vi "KeDSO Initialize Virtual Channels.vi"(8 "error in":errorcluster, 10 "Reset (True)":bool=TRUE, 11 "keysight dso":T1={"VISA"="", "channels"=[], "bw limit [Hz]"=0.0, "resolution"=enum."Basic", "trig noise reject"=enum."Normal", "N"=0, "trigger config"={"trigger source"=enum."Immediate", "trigger slope"=enum."Negative", "level [V]"=0.0, "hysteresis [V]"=0.001, "pre-trig [%]"=50}, "fs [Hz]"=0.0, "timeout stop"=timestamp(0 s since 1904-01-01), "waiting for opc"=FALSE, "fetch offset [smpl]"=0, "abs timestamp"=timestamp(0 s since 1904-01-01), "ranges [V]"=[], "decimation"=0.0, "ext ref"=FALSE, "emulate aperture"=FALSE, "model"=enum."DSO91304"} {"bw limit [Hz]" format="%#_6p"; "channels"."Offset [V]" format="%#_6p"; "channels"."Range [Vpk]" min=0.0 format="%#_6p"; "channels"."Channel" min=1}) -> (0 "error out":errorcluster, 2 "channel ids":string[](array[string]), 3 "keysight dso out":T1={"VISA"="", "channels"=[], "bw limit [Hz]"=0.0, "resolution"=enum."Basic", "trig noise reject"=enum."Normal", "N"=0, "trigger config"={"trigger source"=enum."Immediate", "trigger slope"=enum."Negative", "level [V]"=0.0, "hysteresis [V]"=0.001, "pre-trig [%]"=50}, "fs [Hz]"=0.0, "timeout stop"=timestamp(0 s since 1904-01-01), "waiting for opc"=FALSE, "fetch offset [smpl]"=0, "abs timestamp"=timestamp(0 s since 1904-01-01), "ranges [V]"=[], "decimation"=0.0, "ext ref"=FALSE, "emulate aperture"=FALSE, "model"=enum."DSO91304"} {"bw limit [Hz]" format="%#_6p"; "channels"."Offset [V]" format="%#_6p"; "channels"."Range [Vpk]" min=0.0 format="%#_6p"; "channels"."Channel" min=1})   [LabVIEW 2020]
doc: "Initializes virtual channels of Keysight DSOs according to keysight session data."
uses:
  KeDSO session.ctl
  KeDSO Virtual Channel.ctl
  KeDSO High Resolution Mode.ctl
  KeDSO Trigger Setup.ctl
  KeDSO Trigger Source.ctl
  Agilent 90000 Series.lvlib
  Public/Utility/DSO type.ctl
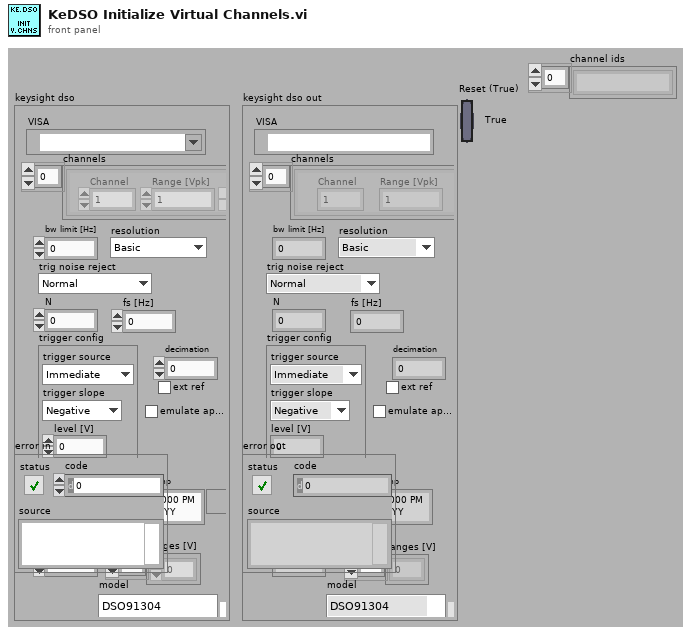
[diagram p1: front panel]
types:
  T1 = typedef "KeDSO session.ctl" = cluster{"VISA":refnum<visa-resource-name>, "channels":T2[], "bw limit [Hz]":dbl, "resolution":T3, "trig noise reject":enum16{"Normal", "High Sensitivity"}, "N":i64, "trigger config":T4, "fs [Hz]":dbl, "timeout stop":timestamp, "waiting for opc":bool, "fetch offset [smpl]":i64, "abs timestamp":timestamp, "ranges [V]":dbl[], "decimation":dbl, "ext ref":bool, "emulate aperture":bool, "model":T6}
  T2 = typedef "KeDSO Virtual Channel.ctl" = cluster{"Channel":i32, "Range [Vpk]":dbl, "btn clr":bool, "btn up":bool, "btn down":bool, "Offset [V]":dbl, "Coupling":enum16{"DC", "DC50", "AC", "LFR1"}, "bw limit enab":bool}
  T3 = typedef "KeDSO High Resolution Mode.ctl" = enum16{"Basic", "High-res AUTO", "Min. 9-bits", "Min. 10-bits", "Min. 11-bits", "Min. 12-bits", "Fixed 11-bits", "Fixed 12-bits", "Fixed 13-bits", "Fixed 14-bits", "Fixed 15-bits", "Fixed 16-bits"}
  T4 = typedef "KeDSO Trigger Setup.ctl" = cluster{"trigger source":T5, "trigger slope":enum16{"Negative", "Positive", "Either"}, "level [V]":dbl, "hysteresis [V]":dbl, "pre-trig [%]":i32}
  T5 = typedef "KeDSO Trigger Source.ctl" = enum16{"Immediate", "Level", "AUX"}
  T6 = typedef "Agilent 90000 Series.lvlib/DSO type.ctl" = enum16{"DSO91304", "DSO91204", "DSO90804", "DSO90604", "DSO90404", "DSO90254", "DSA91304", "DSA91204", "DSA90804", "DSA90604", "DSA90404", "DSA90254", "DSO9104", "DSO9254", "DSO9404", "MSO9104", "MSO9254", "MSO9404", "MSO9064", "DSO9064", "DSOX91604", "DSOX92004", "DSOX92504", "DSOX92804", "DSOX93204", "DSO93004", "DSO9024H", "DSO9054H", "DSO9104H", "DSO9204H", "DSOS054A", "DSOS104A", "DSOS204A", "DSOS254A", "DSOS404A", "DSOS604A", "DSOS804A", "MSOS054A", "MSOS104A", "MSOS204A", "MSOS254A", "MSOS404A", "MSOS604A", "MSOS804A", "DSAX96204Q", "DSOX96204Q", "DSAX95004Q", "DSOX95004Q", "DSAX93304Q", "DSOX93304Q", "DSAX92504Q", "DSOX92504Q", "DSAX92004Q", "DSOX92004Q"}
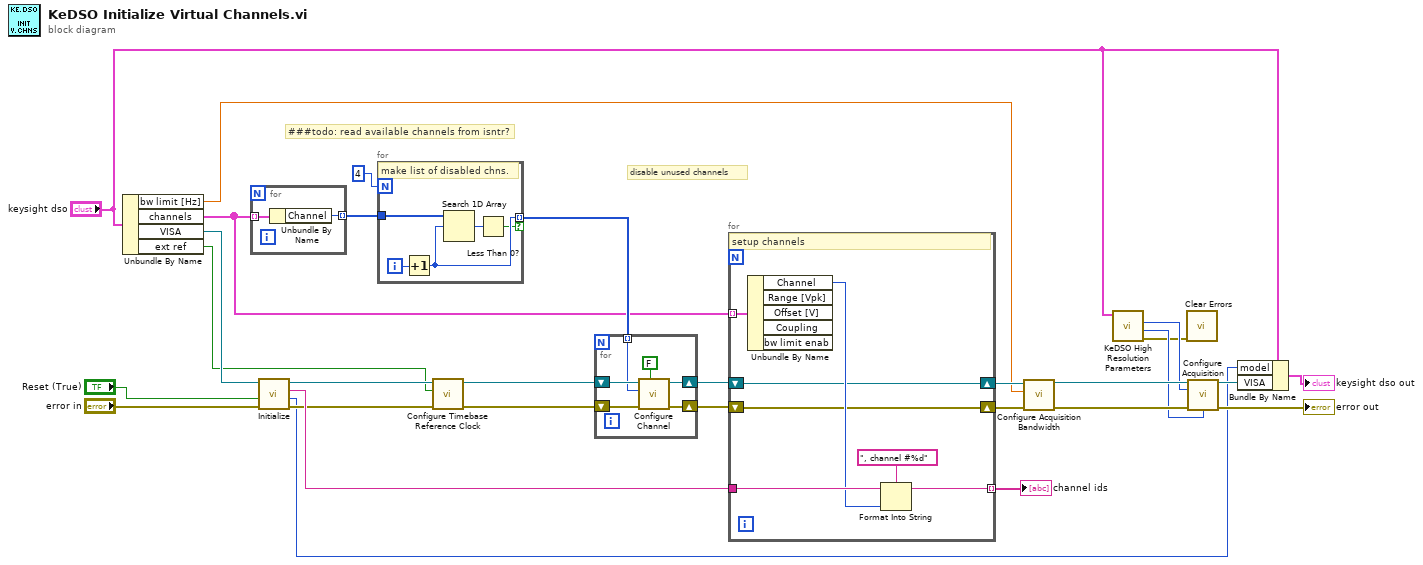
[diagram p0: block diagram]
diagram:
  # "disable unused channels"
  # "###todo: read available channels from isntr?"
  n1 = Unbundle By Name("keysight dso") -> ("bw limit [Hz]"=w18:dbl, "channels"=w21:T2[], "VISA"=w28:refnum<visa-resource-name>, "ext ref"=w2:bool)
  n2 = for {
    tunnel: w21 -> [w31] mode=indexing
    tunnel: [w30] -> w25 mode=indexing
    n3 = Unbundle By Name(w31) -> ("Channel"=w30:i32)
  }
  n4 = call "Initialize.vi"("error in (no error)"="error in", "Reset (True)"="Reset (True)", "VISA resource name"=w28) -> ("error out"=w6:errorcluster, "model"=w1:T6, "idn string"=w16:string, "VISA resource name out"=w5:refnum<visa-resource-name>)  [unwired: 5 in]
  n5 = for {
    N: 4 -> [_]
    tunnel: w25 -> [w36]
    tunnel: [w34] -> w24 mode=indexing if=w32
    i -> [w35]
    # "make list of disabled chns."
    n6 = Increment(x=w35) -> (x+1=w34:i32)
    n7 = Search 1D Array(1D array=w36, element=w34) -> (index of element=w33:i32)  [unwired: 1 in]
    n8 = Less Than 0?(x=w33) -> (x < 0?=w32:bool)
  }
  n9 = call "Configure Timebase Reference Clock.vi"("error in (no error)"=w6, "use ext ref (F: local)"=w2, "VISA resource name"=w5) -> ("error out"=w4:errorcluster, "VISA resource name out"=w3:refnum<visa-resource-name>)  [unwired: 7 in]
  n10 = for {
    shift-right: [w37] -> w22
    shift-left: w3 -> [w41]
    shift-right: [w38] -> w23
    shift-left: w4 -> [w42]
    tunnel: w24 -> [w39] mode=indexing
    n11 = call "Configure Channel.vi"("Enable Channel (T: Enable)"=FALSE, "error in (no error)"=w42, "Channel (1: Channel 1)"=w39, "VISA resource name"=w41) -> ("error out"=w38:errorcluster, "VISA resource name out"=w37:refnum<visa-resource-name>)  [unwired: 6 in]
  }
  n12 = for {
    shift-right: [w44] -> w19
    shift-left: w22 -> [w44]
    shift-right: [w43] -> w20
    shift-left: w23 -> [w43]
    tunnel: w21 -> [w49] mode=indexing
    tunnel: w16 -> [w48]
    tunnel: [w45] -> w15 mode=indexing
    # "setup channels"
    n13 = Unbundle By Name(w49) -> ("Channel"=w46:i32)  [unwired: 4 out]
    n14 = Format Into String(format string=", channel #%d", initial string=w48, w46) -> (resulting string=w45:string)  [unwired: 1 in, 1 out]
  }
  "channel ids" <- w15
  n15 = call "Configure Acquisition Bandwidth.vi"("error in (no error)"=w20, "Acquisition Bandwidth (1000000000)"=w18, "VISA resource name"=w19) -> ("error out"=w12:errorcluster, "VISA resource name out"=w11:refnum<visa-resource-name>)  [unwired: 7 in]
  n16 = call "KeDSO High Resolution Parameters.vi"("keysight dso"="keysight dso") -> ("error out"=w7:errorcluster, "Resolution"=w8:i32, "Acquisition Type"=w9:i32)  [unwired: 4 in, 4 out]
  n17 = call <vilib>:"Clear Errors.vi"("error in (no error)"=w7) -> ()  [unwired: 5 in, 2 out]
  n18 = call "Configure Acquisition.vi"("VISA resource name"=w11, "Acquisition Type (0: Normal)"=w9, "error in (no error)"=w12, "Resolution (0:Auto)"=w8) -> ("VISA resource name out"=w14:refnum<visa-resource-name>, "error out"=→"error out":errorcluster)  [unwired: 10 in]
  n19 = Bundle By Name(cluster="keysight dso", "model"=w1, "VISA"=w14) -> (→"keysight dso out":T1)
